vi "Cleanup Temp Sysdef Files.vi"(6 "bypass cleanup":bool, 8 "error in":errorcluster, 11 "Relative path":path=path "") -> (0 "error out":errorcluster)   [LabVIEW 2017, in "Routing and Faulting System Tests.lvclass"]
uses:
  Routing and Faulting System Tests.lvclass
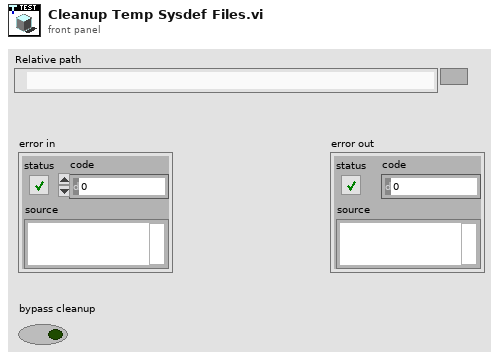
[diagram p1: front panel]
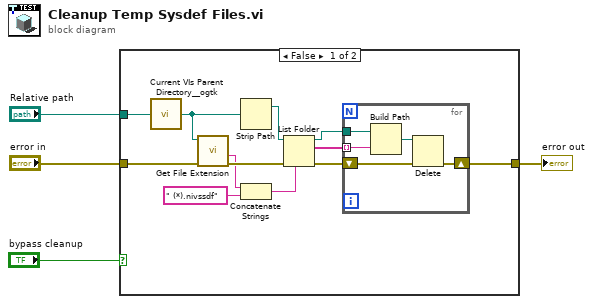
[diagram p0: block diagram]
diagram:
  n1 = case shown="False" "bypass cleanup" {
    tunnel: "Relative path" -> [w16 _]
    tunnel: "error in" -> [w11 w22]
    tunnel: [w5 w22] -> w2
    frame False {
      n2 = call <userlib>:"Current VIs Parent Directory__ogtk.vi"("Relative path (.)"=w16) -> ("Parent Directory (+ Relative)"=w6:path)  [unwired: 4 in]
      n3 = call <vilib>:"Get File Extension.vi"("error in (no error)"=w11, "file"=w6) -> ("error out"=w10:errorcluster, "filename without extension"=w9:string)  [unwired: 5 in, 3 out]
      n4 = Strip Path(path=w6) -> (stripped path=w12:path)  [unwired: 1 out]
      n5 = Concatenate Strings(w9, " (*).nivssdf" ("pattern")) -> (w7:string)
      n6 = List Folder(path=w12, pattern=w7, error in=w10) -> (path out=w15:path, filenames=w14:string[], error out=w13:errorcluster)  [unwired: 1 in, 1 out]
      n7 = for {
        tunnel: w15 -> [w21]
        tunnel: w14 -> [w20] mode=indexing
        shift-right: [w17] -> w5
        shift-left: w13 -> [w18]
        n8 = Build Path(base path=w21, name or relative path=w20) -> (appended path=w19:path)
        n9 = Delete(path (use dialog)=w19, error in=w18) -> (error out=w17:errorcluster)  [unwired: 3 in, 2 out]
      }
    }
    frame True {
    }
  }
  "error out" <- w2
